vi "get queue ref.vi"(8 "error in (no error)":errorcluster, 10 "destination thread":string, 11 "destination app type":T1) -> (0 "error out":errorcluster, 3 "queue ref":refnum<queue>)   [LabVIEW 2012]
uses:
  typedefs/HMI PC thread IDs.ctl
  typedefs/station cDAQ thread IDs.ctl
  typedefs/state queue fglbl actions.ctl
  typedefs/station AuditHMI thread IDs.ctl
  typedefs/interthread message.ctl
  typedefs/app type.ctl
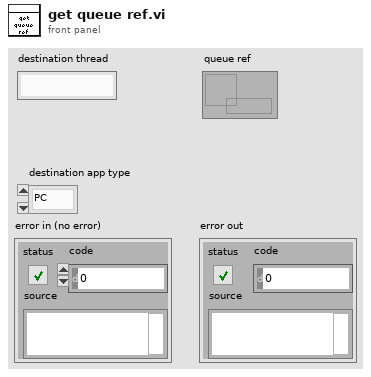
[diagram p1: front panel]
types:
  T1 = typedef "app type.ctl" = enum16{"PC", "cDAQ", "AuditHMI"}
  T2 = typedef "state queue fglbl actions.ctl" = enum16{"init queues", "get queue ref", "destroy queues"}
  T3 = typedef "HMI PC thread IDs.ctl" = enum16{"hmi main", "file output", "tcp comms", "NVH process"}
  T4 = typedef "station AuditHMI thread IDs.ctl" = enum16{"AuditHMI main", "tcp comms"}
  T5 = typedef "station cDAQ thread IDs.ctl" = enum16{"cDAQ main", "analog input", "eol test exe", "nvh test exe", "tcp comms"}
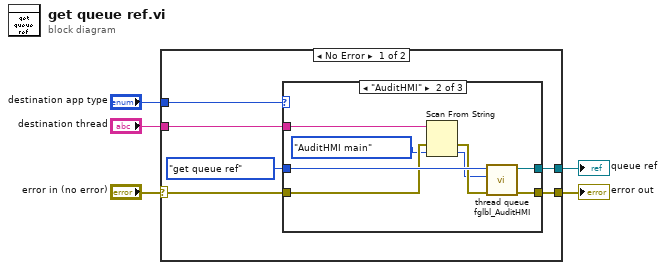
[diagram p0: block diagram]
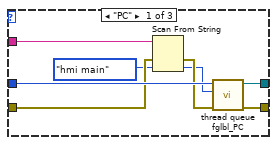
[diagram p2: hidden frame]
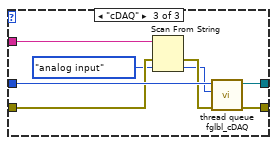
[diagram p3: hidden frame]
diagram:
  n1 = case shown="No Error" "error in (no error)" {
    selector: "error in (no error)" -> [w6 w36]
    tunnel: [w11 w36] -> w5
    tunnel: [w10 _] -> w4
    tunnel: "destination app type" -> [w9 _]
    tunnel: "destination thread" -> [w8 _]
    frame No Error {
      n2 = case shown="\"AuditHMI\"" w9 {
        tunnel: state_queue_fglbl_actions."get queue ref" ("action") -> [w19 w27 w35]
        tunnel: [w18 w26 w34] -> w10
        tunnel: [w17 w25 w33] -> w11
        tunnel: w6 -> [w16 w24 w32]
        tunnel: w8 -> [w13 w22 w28]
        frame "PC" {
          n3 = Scan From String(input string=w13, error in=w16, default 1=HMI_PC_thread_IDs."hmi main" ("PC HMI Thread Queues")) -> (error out=w15:errorcluster, output 1=w12:T3)  [unwired: 2 in, 2 out]
          n4 = call "thread queue fglbl_PC.vi"("error in (no error)"=w15, "Station cDAQ Thread Queue"=w12, "action"=w19) -> ("error out"=w17:errorcluster, "queue out"=w18:refnum<queue>)  [unwired: 6 in, 1 out]
        }
        frame "AuditHMI" {
          n5 = Scan From String(input string=w22, error in=w24, default 1=station_AuditHMI_thread_IDs."AuditHMI main" ("Station AuditHMI Thread ID")) -> (error out=w23:errorcluster, output 1=w20:T4)  [unwired: 2 in, 2 out]
          n6 = call "thread queue fglbl_AuditHMI.vi"("error in (no error)"=w23, "Station AuditHMI Thread ID"=w20, "action"=w27) -> ("error out"=w25:errorcluster, "queue out"=w26:refnum<queue>)  [unwired: 6 in, 1 out]
        }
        frame "cDAQ" {
          n7 = Scan From String(input string=w28, error in=w32, default 1=station_cDAQ_thread_IDs."analog input" ("Station cDAQ Thread Queues")) -> (error out=w31:errorcluster, output 1=w29:T5)  [unwired: 2 in, 2 out]
          n8 = call "thread queue fglbl_cDAQ.vi"("error in (no error)"=w31, "Station cDAQ Thread Queue"=w29, "action"=w35) -> ("error out"=w33:errorcluster, "queue out"=w34:refnum<queue>)  [unwired: 6 in, 1 out]
        }
      }
    }
    frame Error {
    }
  }
  "error out" <- w5
  "queue ref" <- w4
